vi "Set Digital Inputs.vi"(8 "error in (no error)":errorcluster, 10 "State":bool, 11 "Stage Actor.lvlib:Stage.lvclass":refnum<class "Stage.lvclass">) -> (0 "error out":errorcluster, 3 "Stage Actor.lvlib:Stage.lvclass 2":refnum<class "Stage.lvclass">)   [LabVIEW 2018, in "Stage Actor.lvlib" / "Stage.lvclass"]
uses:
  Stage.lvclass
  Stage.lvclass/Stage.ctl
  <vilib>/DAQmx/write.llb/DAQmx Write (Digital Bool 1Line 1Point).vi
  <vilib>/DAQmx/miscellaneous.llb/DAQmx Fill In Error Info.vi
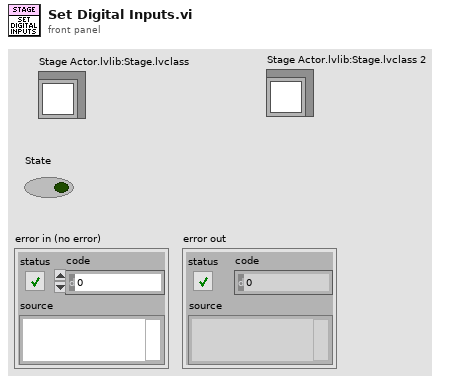
[diagram p1: front panel]
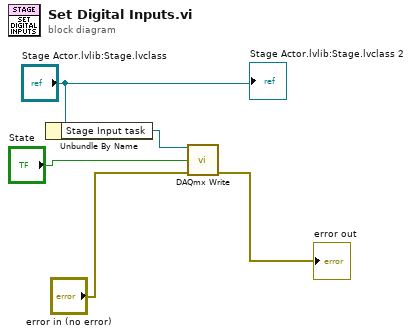
[diagram p0: block diagram]
diagram:
  n1 = Unbundle By Name("Stage Actor.lvlib:Stage.lvclass") -> ("Stage Input task"=w5:refnum<k21>)
  n2 = call-poly <vilib>:"DAQmx Write.vi"("task/channels in"=w5, "data"="State", "error in"="error in (no error)") -> ("error out"=→"error out":errorcluster)  [unwired: 10 in, 2 out]
  "Stage Actor.lvlib:Stage.lvclass 2" <- "Stage Actor.lvlib:Stage.lvclass"
